vi "Intan_resetTeensy.vi"() -> ()   [LabVIEW 2011]
panel:
  out "read buffer":string
  out "Text response":string
  in  "Nbytes initial response":u32=72
  in  "VISA resource name":refnum<visa-resource-name>="COM3"
  out "error out":errorcluster
  in  "error in":errorcluster
  out "status 2":bool
  out "i 2":i32
  in  "stop 2":bool
  out "code 2":i32
  out "code":i32
  in  "stop":bool
  out "i":i32
  out "status":bool
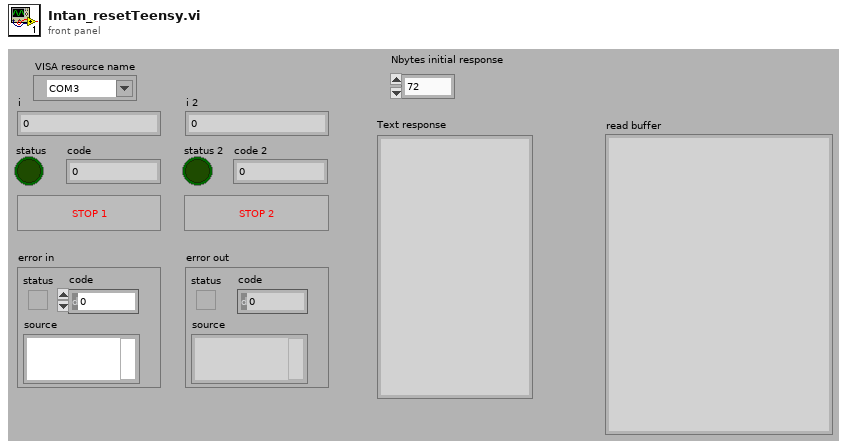
[diagram p1: front panel]
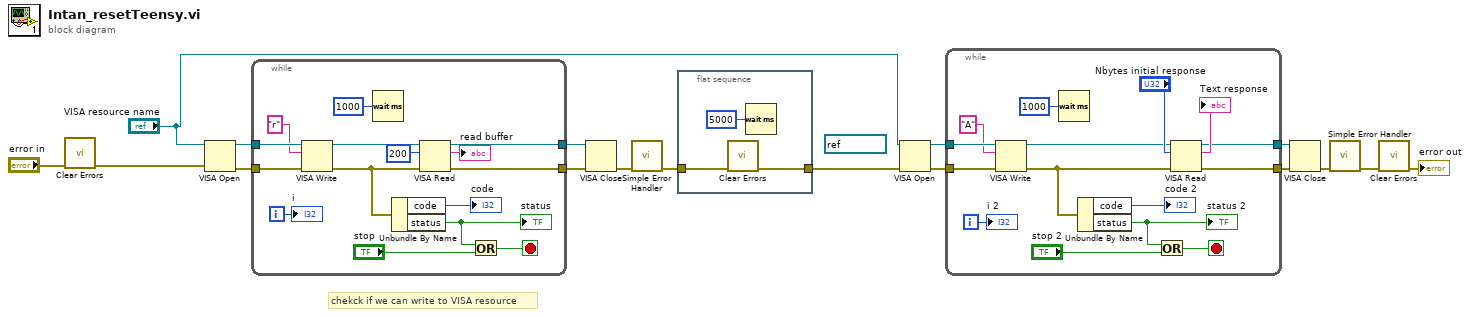
[diagram p0: block diagram]
diagram:
  (unwired) refnum<visa-resource-name> "COM3" ("VISA resource name")
  # "chekck if we can write to VISA resource"
  n1 = call <vilib>:"Clear Errors.vi"("error in (no error)"="error in") -> ("error out"=w6:errorcluster)  [unwired: 6 in]
  n2 = VISA Open(error in (no error)=w6, VISA resource name="VISA resource name") -> (VISA resource name=w14:refnum<visa-resource-name>, error out=w16:errorcluster)  [unwired: 3 in]
  n3 = while {
    tunnel: [w20] -> w17
    tunnel: w16 -> [w29]
    tunnel: [w21] -> w15
    tunnel: w14 -> [w30]
    i -> [w31]
    stop <- w26 stop-if-true
    n4 = VISA Write(VISA resource name=w30, write buffer="r", error in (no error)=w29) -> (VISA resource name out=w23:refnum<visa-resource-name>, error out=w22:errorcluster)  [unwired: 1 out]
    n5 = Wait (ms)(milliseconds to wait=u32 1000) -> ()  [unwired: 1 out]
    n6 = Unbundle By Name(w22) -> ("code"=→"code":i32, "status"=w28:bool)
    "status" <- w28
    n7 = VISA Read(VISA resource name=w23, byte count=u32 200, error in (no error)=w22) -> (VISA resource name out=w21:refnum<visa-resource-name>, read buffer=→"read buffer":string, error out=w20:errorcluster)  [unwired: 1 out]
    n8 = Or(x=w28, y="stop") -> (x .or. y?=w26:bool)
    "i" <- w31
  }
  n9 = VISA Close(VISA resource name=w15, error in (no error)=w17) -> (error out=w13:errorcluster)
  n10 = call <vilib>:"Simple Error Handler.vi"("error in (no error)"=w13) -> ("error out"=w12:errorcluster)  [unwired: 4 in, 4 out]
  n11 = flat-sequence {
    tunnel: w12 -> [w34]
    tunnel: [w33] -> w11
    frame #0 {
      n12 = call <vilib>:"Clear Errors.vi"("error in (no error)"=w34) -> ("error out"=w33:errorcluster)  [unwired: 6 in]
      n13 = Wait (ms)(milliseconds to wait=u32 5000) -> ()  [unwired: 1 out]
    }
  }
  n14 = VISA Open(error in (no error)=w11, VISA resource name="VISA resource name") -> (VISA resource name=w9:refnum<visa-resource-name>, error out=w10:errorcluster)  [unwired: 3 in]
  n15 = while {
    tunnel: [w37] -> w7
    tunnel: w10 -> [w47]
    tunnel: w9 -> [w48]
    tunnel: [w36] -> w1
    i -> [w49]
    stop <- w44 stop-if-true
    n16 = VISA Write(VISA resource name=w48, write buffer="A", error in (no error)=w47) -> (VISA resource name out=w39:refnum<visa-resource-name>, error out=w38:errorcluster)  [unwired: 1 out]
    n17 = Wait (ms)(milliseconds to wait=u32 1000) -> ()  [unwired: 1 out]
    n18 = Unbundle By Name(w38) -> ("code"=→"code 2":i32, "status"=w46:bool)
    "status 2" <- w46
    n19 = Or(x=w46, y="stop 2") -> (x .or. y?=w44:bool)
    n20 = VISA Read(VISA resource name=w39, byte count="Nbytes initial response", error in (no error)=w38) -> (VISA resource name out=w36:refnum<visa-resource-name>, read buffer=→"Text response":string, error out=w37:errorcluster)  [unwired: 1 out]
    "i 2" <- w49
  }
  n21 = VISA Close(VISA resource name=w1, error in (no error)=w7) -> (error out=w8:errorcluster)
  n22 = call <vilib>:"Simple Error Handler.vi"("error in (no error)"=w8) -> ("error out"=w4:errorcluster)  [unwired: 4 in, 4 out]
  n23 = call <vilib>:"Clear Errors.vi"("error in (no error)"=w4) -> ("error out"=→"error out":errorcluster)  [unwired: 6 in]
